vi "Channel States json test.vi"() -> ()   [LabVIEW 2017, in "Switch Scripting.lvlib"]
uses:
  Switch Scripting.lvlib
  Channel States.ctl
  Routing State.ctl
  Routing Channel/Connection.ctl
panel:
  out "Channel States from JSON":T1=[{"name"="", "value"=23, "Connection List"=[{"Source"="2010A:J1Ch0p", "Destination"="2010A:J2Ch16p"}]}, {"name"="", "value"=34, "Connection List"=[{"Source"="2010A:J1Ch0p", "Destination"="2010A:J2Ch0p"}, {"Source"="2010B:J1Ch0p", "Destination"="2010B:J2Ch0p"}]}]
  out "Connection List":cluster{"Source":string, "Destination":string}[](array[cluster])
  in  "run-time Channel state":i32
  out "Property: Channel State Lookup (Compiled?)":i32[](array[numeric])
  out "JSON string":string
  in  "Channel States":T1=[{"name"="", "value"=23, "Connection List"=[{"Source"="2010A:J1Ch0p", "Destination"="2010A:J2Ch16p"}]}, {"name"="", "value"=34, "Connection List"=[{"Source"="2010A:J1Ch0p", "Destination"="2010A:J2Ch0p"}, {"Source"="2010B:J1Ch0p", "Destination"="2010B:J2Ch0p"}]}]
  # "Compiled --- >>"
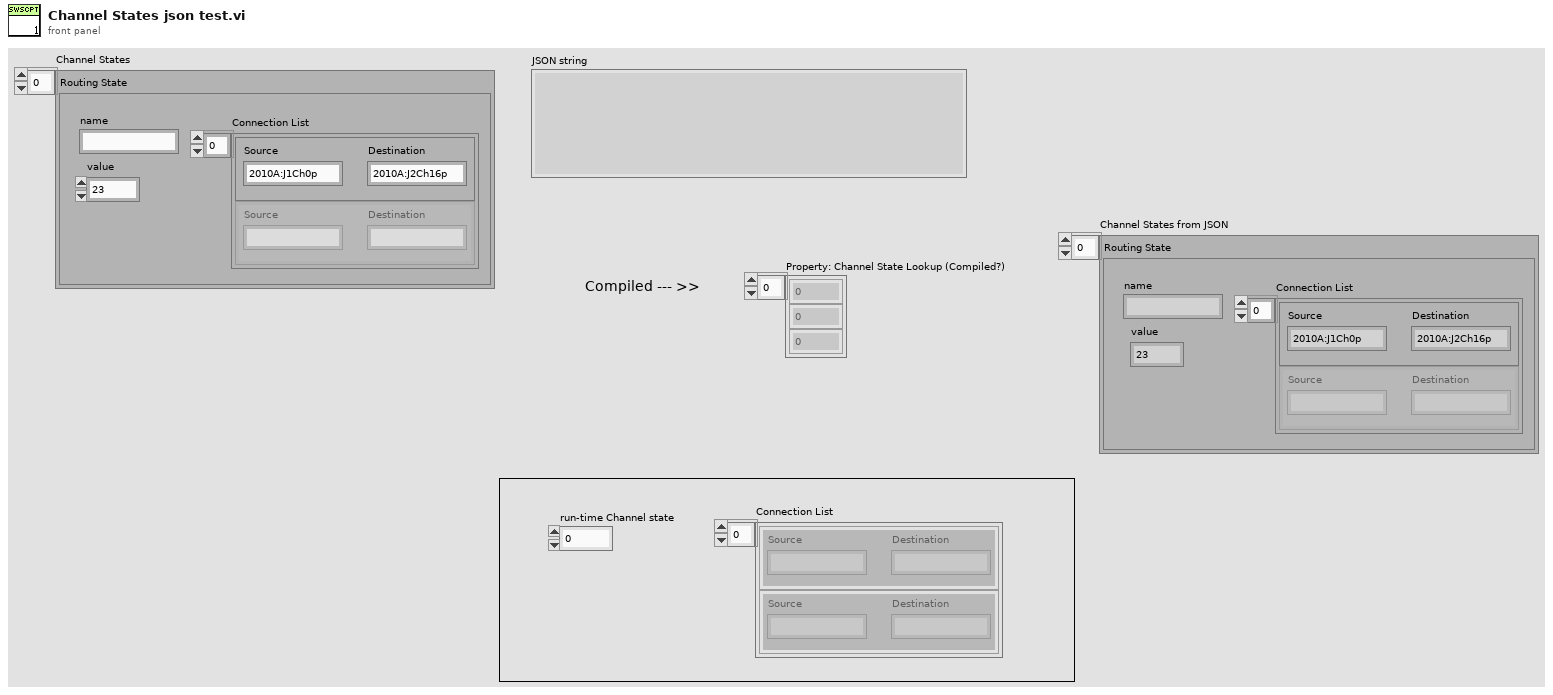
[diagram p1: front panel]
types:
  T1 = typedef "Switch Scripting.lvlib/Channel States.ctl" = T2[]
  T2 = typedef "Switch Scripting.lvlib/Routing State.ctl" = cluster{"name":string, "value":i32, "Connection List":T3[]}
  T3 = typedef "Switch Scripting.lvlib/Connection.ctl" = cluster{"Source":string, "Destination":string}
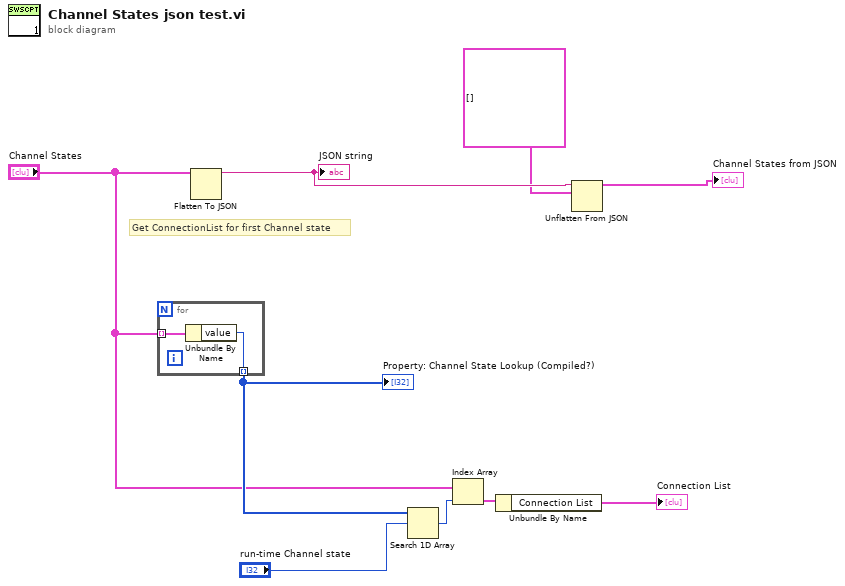
[diagram p0: block diagram]
diagram:
  # "Get ConnectionList for first Channel state"
  n1 = for {
    tunnel: "Channel States" -> [w11] mode=indexing
    tunnel: [w10] -> w8 mode=indexing
    n2 = Unbundle By Name(w11) -> ("value"=w10:i32)
  }
  "Property: Channel State Lookup (Compiled?)" <- w8
  n3 = Flatten To JSON(anything="Channel States") -> (JSON string=w4:string)  [unwired: 2 in, 1 out]
  "JSON string" <- w4
  n4 = Search 1D Array(1D array=w8, element="run-time Channel state") -> (index of element=w6:i32)  [unwired: 1 in]
  n5 = Index Array(array="Channel States", index=w6) -> (element=w9:T2)
  n6 = Unbundle By Name(w9) -> ("Connection List"=→"Connection List":T3[])
  n7 = Unflatten From JSON(JSON string=w4, type and defaults=T1 [] ("Channel States")) -> (value=→"Channel States from JSON":T1)  [unwired: 5 in, 1 out]
